vi "upper_lower_case.vi"() -> ()   [LabVIEW 2019]
panel:
  out "all lower case string 2":string
  out "all upper case string":string
  out "all lower case string":string
  in  "String 3":string="Ashutosh"
  in  "String 2":string="ASHUTOSH"
  in  "String":string="ashutosh"
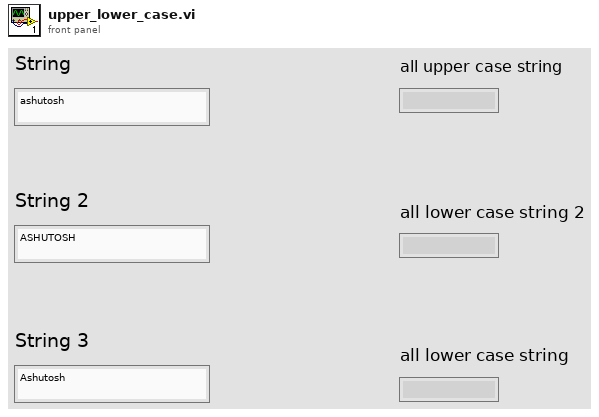
[diagram p1: front panel]
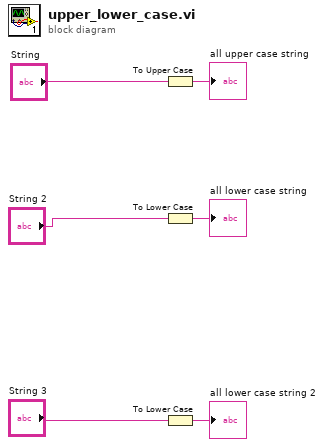
[diagram p0: block diagram]
diagram:
  n1 = To Upper Case(1:"String") -> (0:→"all upper case string":string)
  n2 = To Lower Case(string="String 2") -> (all lower case string=→"all lower case string":string)
  n3 = To Lower Case(string="String 3") -> (all lower case string=→"all lower case string 2":string)
